vi "Station Read Station Initialize file.vi"(8 "error in (no error)":errorcluster, 11 "Station in":refnum<class "Station.lvclass">) -> (0 "error out":errorcluster, 3 "Station out":refnum<class "Station.lvclass">)   [LabVIEW 2018, in "Station.lvclass"]
uses:
  Station.lvclass
  Station.lvclass/Station.ctl
  <vilib>/Utility/file.llb/Read From Spreadsheet File (string).vi
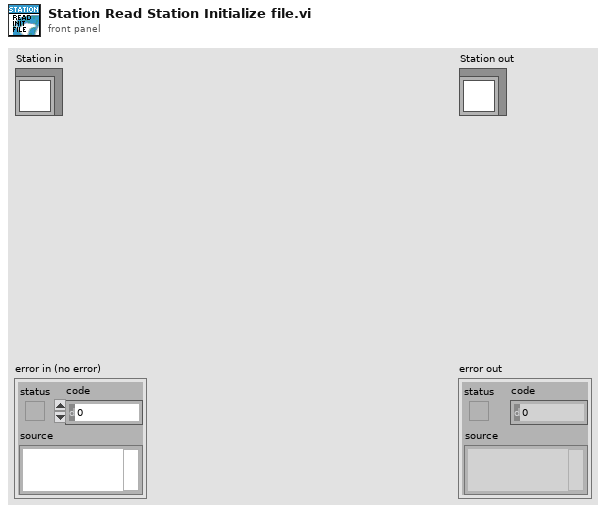
[diagram p1: front panel]
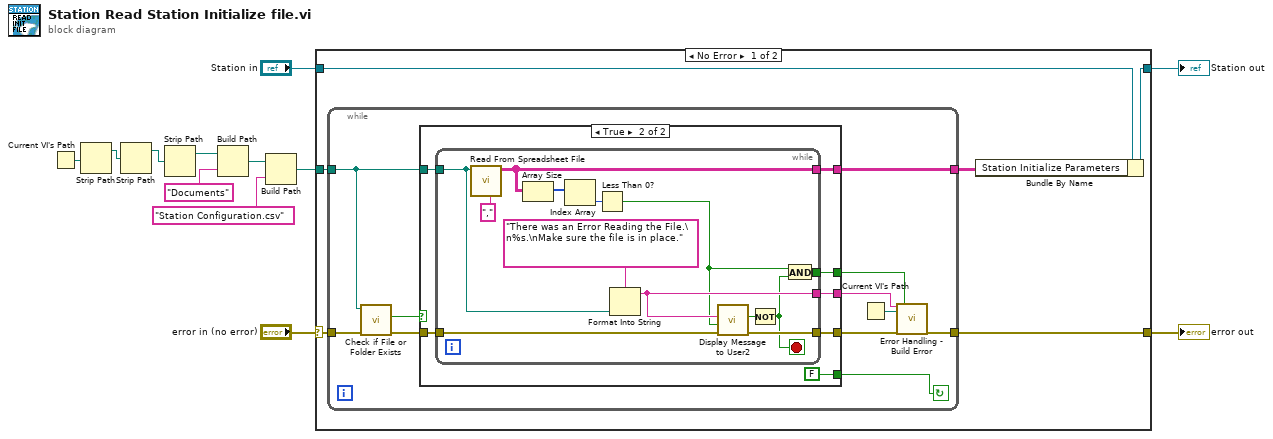
[diagram p0: block diagram]
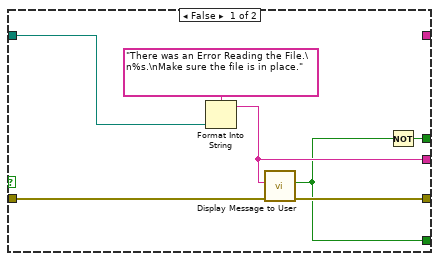
[diagram p2: hidden frame]
diagram:
  n1 = Current VI's Path() -> (path=w12:path)
  n2 = Strip Path(path=w12) -> (stripped path=w2:path)  [unwired: 1 out]
  n3 = Strip Path(path=w2) -> (stripped path=w1:path)  [unwired: 1 out]
  n4 = Strip Path(path=w1) -> (stripped path=w10:path)  [unwired: 1 out]
  n5 = Build Path(base path=w10, name or relative path="Documents") -> (appended path=w8:path)
  n6 = Build Path(base path=w8, name or relative path="Station Configuration.csv") -> (appended path=w7:path)
  n7 = case shown="No Error" "error in (no error)" {
    selector: "error in (no error)" -> [w18 w58]
    tunnel: [w16 w58] -> w5
    tunnel: w7 -> [w17 _]
    tunnel: "Station in" -> [w15 w57]
    tunnel: [w14 w57] -> w3
    frame No Error {
      n8 = while {
        tunnel: [w29] -> w13
        tunnel: w17 -> [w26]
        tunnel: w18 -> [w28]
        tunnel: [w21] -> w16
        stop <- w24 continue-if-true
        n9 = call <vilib>:"Check if File or Folder Exists.vi"("error in (no error)"=w28, "path"=w26) -> ("error out"=w27:errorcluster, "file or folder exists?"=w25:bool)  [unwired: 7 in, 1 out]
        n10 = case shown="True" w25 {
          tunnel: [_ w43] -> w29
          tunnel: [w35 w39] -> w22
          tunnel: w27 -> [w36 w42]
          tunnel: w26 -> [w33 w41]
          tunnel: [w30 FALSE ("OK")] -> w24
          tunnel: [w31 w38] -> w20
          tunnel: [w32 w37] -> w19
          frame False {
            n11 = Format Into String(format string="There was an Error Reading the File.\n%s.\nMake sure the file is in place." ("Error Message"), w33) -> (resulting string=w32:string)  [unwired: 2 in, 1 out]
            n12 = call "Display Message to User"("error in (no error)"=w36, "Message"=w32) -> ("error out"=w35:errorcluster, "REPEAT"=w30:bool)  [unwired: 8 in]
            n13 = Not(x=w30) -> (.not. x?=w31:bool)
          }
          frame True {
            n14 = while {
              tunnel: [w55] -> w43
              tunnel: w41 -> [w51]
              tunnel: w42 -> [w50]
              tunnel: [w49] -> w39
              tunnel: [w47] -> w37
              tunnel: [w44] -> w38
              stop <- w46 stop-if-true
              n15 = call-poly <vilib>:"Read From Spreadsheet File.vi"("delimiter (\\t)"="," ("delimiter (\\t)"), "file path (dialog if empty)"=w51) -> ("all rows"=w55:string[][])  [unwired: 5 in, 4 out]
              n16 = Array Size(array=w55) -> (size(s)=w54:i32[])
              n17 = Index Array(array=w54) -> (element=w53:i32)  [unwired: 1 in]
              n18 = Less Than 0?(x=w53) -> (x < 0?=w45:bool)
              n19 = Format Into String(format string="There was an Error Reading the File.\n%s.\nMake sure the file is in place." ("Error Message"), w51) -> (resulting string=w47:string)  [unwired: 2 in, 1 out]
              n20 = call "Display Message to User2"("error in (no error)"=w50, "Enable"=w45, "Message"=w47) -> ("error out"=w49:errorcluster, "Repeat"=w48:bool)  [unwired: 7 in]
              n21 = Not(x=w48) -> (.not. x?=w46:bool)
              n22 = And(x=w45, y=w46) -> (x .and. y?=w44:bool)
            }
          }
        }
        n23 = Current VI's Path() -> (path=w23:path)
        n24 = call "Error Handling - Build Error.vi"("Error Message"=w19, "VI Path (calling VI path)"=w23, "error in (no error)"=w22, "Create Error? (T)"=w20) -> ("error out"=w21:errorcluster)  [unwired: 15 in]
      }
      n25 = Bundle By Name(cluster=w15, "Station Initialize Parameters"=w13) -> (w14:refnum<class "Station.lvclass">)
    }
    frame Error {
    }
  }
  "error out" <- w5
  "Station out" <- w3
